vi "Double FFT Mesurament (Max Bin detection - Control - Init Wave&Window - Snapshot - DoubleFFT - Latency - Low Freq) RT Test.vi"() -> ()   [LabVIEW 2014]
uses:
  <vilib>/Platform/TimedLoop/XDataNode/timing_clust.ctl
  <vilib>/Platform/TimedLoop/XDataNode/nitl_modes.ctl
  <vilib>/Platform/TimedLoop/XDataNode/wakeup.ctl
  <vilib>/FPGAPlugInAG/sbRIO-9636/niLvFpga_Open_sbRIO-9636.vi
  <vilib>/rvi/interface/common/dynamic/niFpgaDynamicAddResources.vi
  <vilib>/Utility/error.llb/Error Cluster From Error Code.vi
  <vilib>/rvi/errors/niLvFpgaAdjustHostInterfaceError.vi
  <vilib>/rvi/interface/common/niFpgaWaitOnOcc.vi
  <vilib>/FPGAPlugInAG/Dynamic/niLvFpga_Run_Dynamic.vi
  <vilib>/FPGAPlugInAG/Dynamic/niLvFpga_Abort_Dynamic.vi
  <vilib>/FPGAPlugInAG/Dynamic/niLvFpga_Reset_Dynamic.vi
  <vilib>/FPGAPlugInAG/Dynamic/niLvFpga_Close_Dynamic.vi
  <vilib>/rvi/interface/nirviOpenFPGA/nirviOpenFPGA.xnode
  FPGA Bitfiles/LaserDistanceSen_FPGATarget_DoubleFFTMesuram_ltZoZsQg6NE.lvbitx
  FPGA Target/Test VIs/Double FFT Mesurament (Max Bin detection - Control - Init Wave&Window - Snapshot - DoubleFFT - Latency - Low Freq) test.vi
  <vilib>/rvi/interface/nirviReadWriteControl/nirviReadWriteControl.xnode
  <vilib>/rvi/interface/nirviMethod/nirviMethod.xnode
  <vilib>/Platform/TimedLoop/XDataNode/XDataNode.xnode
  <vilib>/rvi/interface/nirviCloseFPGA/nirviCloseFPGA.xnode
  <vilib>/FPGAPlugInAG/Dynamic/niLvFpga_ConfigureFifo_Dynamic.vi
  <vilib>/rvi/errors/niLvFpgaMergeErrorWithErrorCode.vi
  <vilib>/FPGAPlugInAG/Dynamic/niLvFpga_StartFifo_Dynamic.vi
  <vilib>/rvi/interface/Simulation/niFpgaSimulationCallBeginRW.vi
  <vilib>/FPGAPlugInAG/Dynamic/niLvFpga_ReadFifo_Dynamic.vi
  <vilib>/Platform/TimedLoop/XDataNode/XDNodeRunTimeDep.lvlib
  NiFpgaLv.dll
panel:
  out "maxbin_secondFFT":i32
  out "maxbin_firstFFT":i32
  out "F_rise":dbl
  out "f_fall":dbl
  out "f_mean":dbl
  out "Velocity (m/s)":dbl
  out "Distance (m)":dbl
  in  "Initial Latency points":u32(slide)=10 scale=0.0..1249.0
  out "Second FFT (bin)":dbl[](graph)
  out "Second Signal (points) - Rising Triangular":dbl[](graph)
  out "Elements Remaining FFT":u32
  out "Elements Remaining Signal":u32
  out "First FFT (bin)":dbl[](graph)
  out "First Signal (points) - Falling Triangular":dbl[](graph)
  in  "Snapshot":bool
  in  "Windowing":T1(ring)
  in  "first bin":i32=15
  in  "last bin":i32=255
  in  "lower limit 2":u32(slide)=725 scale=625.0..738.0
  in  "lower limit 1":u32(slide)=100 scale=0.0..113.0
  out "Detected Frequency Tone - (Hz)":dbl
  in  "stop":bool
  out "Max Bin":i32
  out "Max Amp":dbl format="%.2f"
  out "Prev Bin":i32
  out "Next Bin":i32
  out "Prev Amp":dbl format="%.2f"
  out "Next Amp":dbl format="%.2f"
  out "Interpolated Bin":dbl
  in  "Interpolation Method":T2(ring)=enum."Jain"
  # "WARNING:\nOnce pressed wait untill the end of operation"
  # "ONLINE parameter"
  # "OFFLINE parameters"
  # "Max Detection FFT bin range"
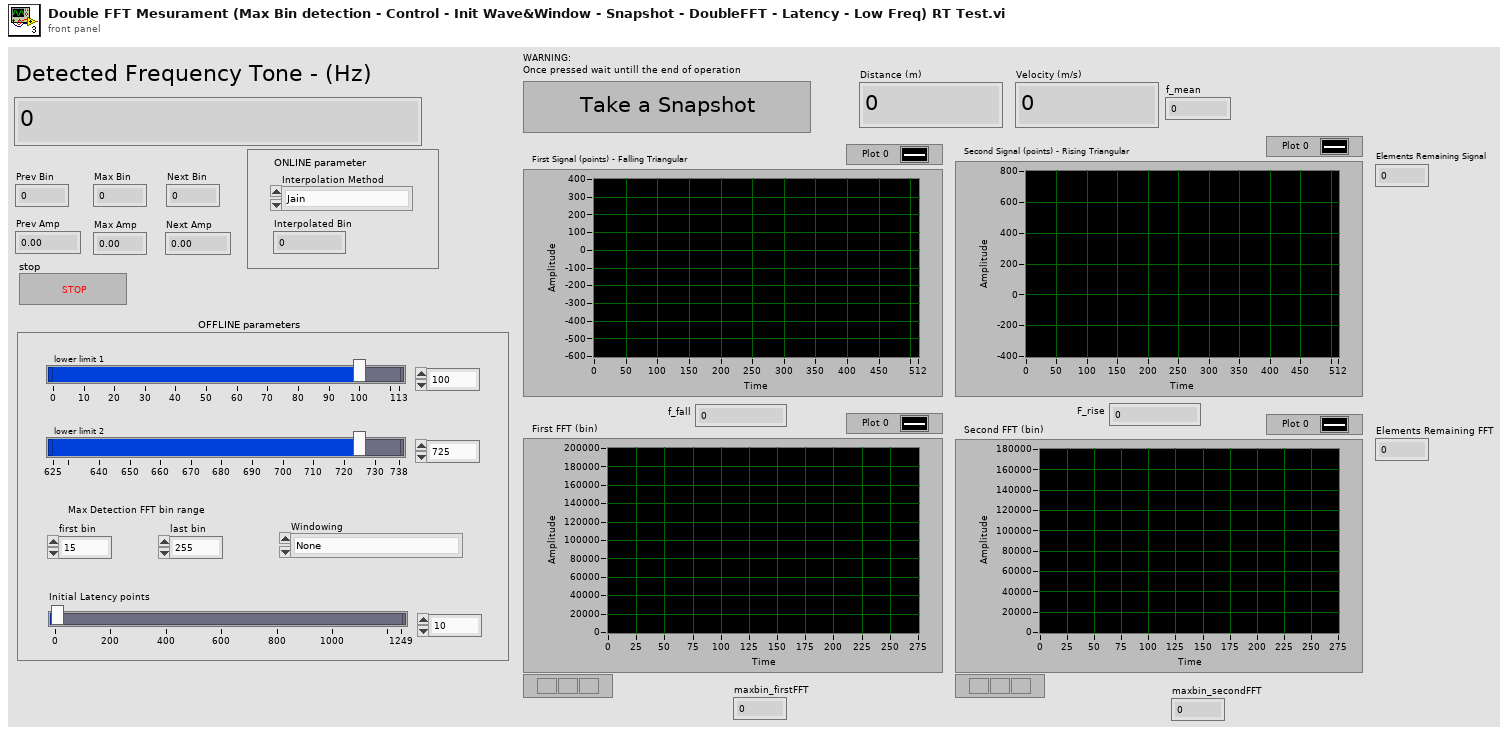
[diagram p1: front panel]
types:
  T1 = enum16{"None", "Hanning", "Hamming", "Blackman", "Blackman-Harris"}
  T2 = enum16{"Quadratic", "McLeodd", "Barycentric", "Jain"}
  T3 = typedef "XDNodeRunTimeDep.lvlib/timing_clust.ctl" = cluster{"Expected End [f-1]":u64, "Actual End [f-1]":u64, "Finished Late? [f-1]":bool, "Expected End [i-1]":u64, "Actual End [i-1]":u64, "Finished Late? [i-1]":bool, "Expected Start [i]":u64, "Actual Start [i]":u64, "Expected Start [f]":u64, "Actual Start [f]":u64, "Source Name":string, "Structure Name":string, "Period":i64, "Deadline":i64, "Offset":i64, "Start":i64, "Priority":i32, "Timeout":i32, "Mode":T4, "Wakeup Reason":T5, "Error":errorcluster, "Source Type":string, "Secondary Source Type":string, "Global End Time":u64, "Global Start Time":u64, "Frame Duration":u64, "Iteration Duration":u64, "Assigned CPU":i32, "I/O Scan Engine Mode":u32}
  T4 = typedef "XDNodeRunTimeDep.lvlib/nitl_modes.ctl" = enum32{"No Change", "Process missed periods, maintain original phase", "Discard missed periods, maintain original phase", "Process missed periods, ignore original phase", "Discard missed periods, ignore original phase"}
  T5 = typedef "XDNodeRunTimeDep.lvlib/wakeup.ctl" = enum32{"Normal", "Aborted", "Asynchronous wakeup", "Timing source error", "Timed loop error", "Timeout"}
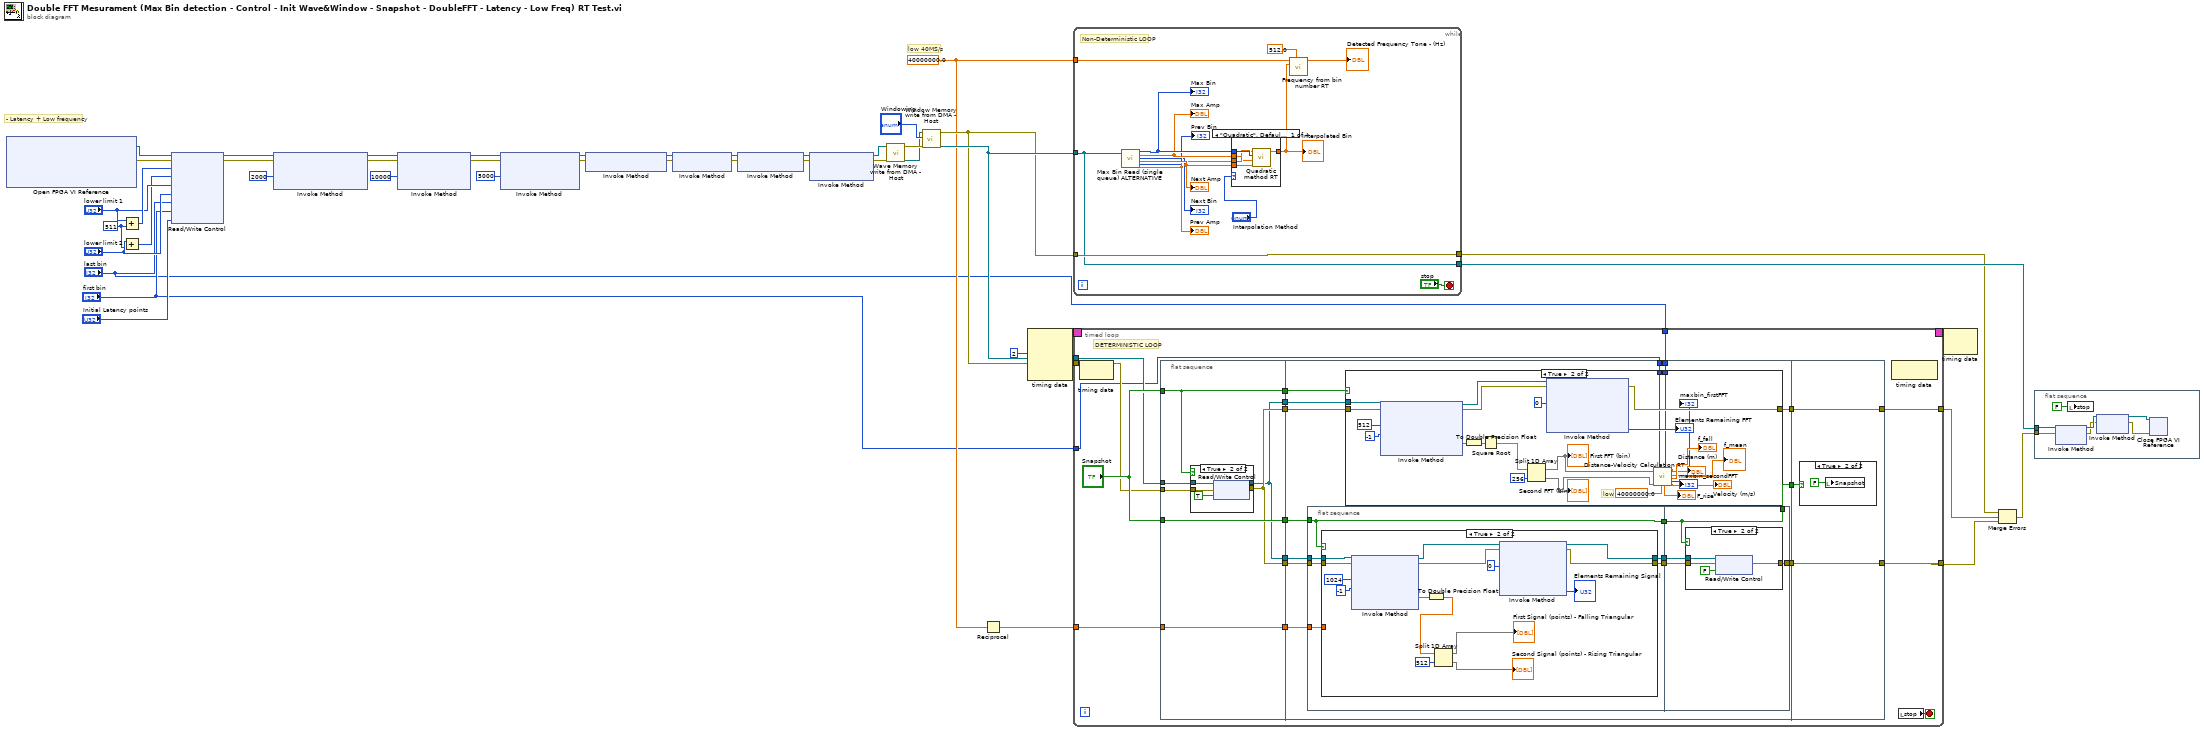
[diagram p0: block diagram]
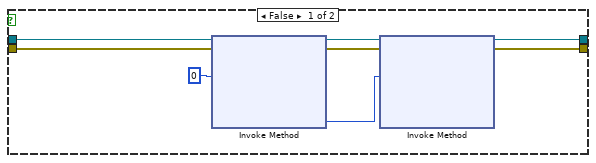
[diagram p3: hidden frame]
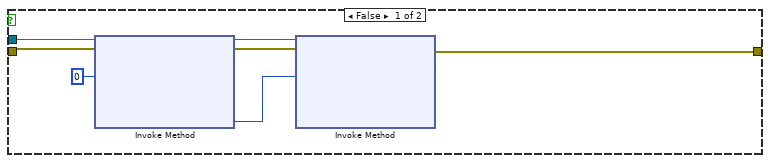
[diagram p5: hidden frame]
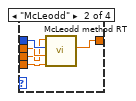
[diagram p7: hidden frame]
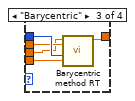
[diagram p8: hidden frame]
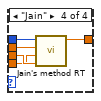
[diagram p9: hidden frame]
diagram:
  w40 = u32 511 ("y")
  w18 = 40000000.0 ("Sample Rate (S/s)")
  # "- Latency + Low frequency"
  # "low 40MS/s"
  n1 = xnode "Open FPGA VI Reference"() -> ("FPGA VI Reference Out"=w39:refnum<k20>, "error out"=w38:errorcluster)  [unwired: 2 in]
  n2 = Add(x="lower limit 1", y=w40) -> (x+y=w44:u32)
  n3 = Add(x="lower limit 2", y=w40) -> (x+y=w42:u32)
  n4 = xnode "Read/Write Control"("FPGA VI Reference In"=w39, "error in"=w38, "upper limit 1"=w44, "upper limit 2"=w42, "lower limit 1"="lower limit 1", "lower limit 2"="lower limit 2", "last bin"="last bin", "first bin"="first bin", "Latency points"="Initial Latency points") -> ("FPGA VI Reference Out"=w33:refnum<k20>, "error out"=w32:errorcluster)
  n5 = xnode "Invoke Method"("FPGA VI Reference In"=w33, "error in"=w32, "Requested Depth"=u32 2000) -> ("FPGA VI Reference Out"=w31:refnum<k20>, "error out"=w30:errorcluster)  [unwired: 1 out]
  n6 = xnode "Invoke Method"("FPGA VI Reference In"=w31, "error in"=w30, "Requested Depth"=u32 10000) -> ("FPGA VI Reference Out"=w29:refnum<k20>, "error out"=w28:errorcluster)  [unwired: 1 out]
  n7 = xnode "Invoke Method"("FPGA VI Reference In"=w29, "error in"=w28, "Requested Depth"=u32 5000) -> ("FPGA VI Reference Out"=w12:refnum<k20>, "error out"=w13:errorcluster)  [unwired: 1 out]
  n8 = xnode "Invoke Method"("FPGA VI Reference In"=w12, "error in"=w13) -> ("FPGA VI Reference Out"=w22:refnum<k20>, "error out"=w21:errorcluster)
  n9 = xnode "Invoke Method"("FPGA VI Reference In"=w22, "error in"=w21) -> ("FPGA VI Reference Out"=w24:refnum<k20>, "error out"=w23:errorcluster)
  n10 = xnode "Invoke Method"("FPGA VI Reference In"=w24, "error in"=w23) -> ("FPGA VI Reference Out"=w10:refnum<k20>, "error out"=w11:errorcluster)
  n11 = xnode "Invoke Method"("FPGA VI Reference In"=w10, "error in"=w11) -> ("FPGA VI Reference Out"=w17:refnum<k20>, "error out"=w16:errorcluster)  [unwired: 1 in]
  n12 = call "Wave Memory write from DMA - Host.vi"("error in"=w16, "FPGA VI Reference In"=w17) -> ("FPGA VI Reference Out"=w14:refnum<k20>, "error out"=w15:errorcluster)  [unwired: 7 in, 1 out]
  n13 = call "Window Memory write from DMA - Host.vi"("error in"=w15, "Enum"="Windowing", "FPGA VI Reference In"=w14) -> ("FPGA VI Reference Out"=w35:refnum<k20>, "error out"=w34:errorcluster)  [unwired: 5 in, 2 out]
  n14 = Reciprocal(x=w18) -> (1/x=w19:dbl)
  n15 = node-c288(i64 2 ("Period")) -> (w9:T3)  [unwired: 3 in]
  n16 = while {
    tunnel: w18 -> [w57]
    tunnel: w35 -> [w55]
    tunnel: w34 -> [w56]
    tunnel: [w55] -> w37
    tunnel: [w56] -> w5
    stop <- "stop" stop-if-true
    # "Non-Deterministic LOOP"
    n17 = call "Max Bin Read (single queue) ALTERNATIVE.vi"("FPGA VI Reference In"=w55) -> ("Max Bin"=w51:i32, "Max Amp"=w50:dbl, "Next Bin"=→"Next Bin":i32, "Next Amp"=w49:dbl, "Prev Bin"=→"Prev Bin":i32, "Prev Amp"=w48:dbl)  [unwired: 12 in, 1 out]
    "Max Bin" <- w51
    "Max Amp" <- w50
    "Prev Amp" <- w48
    "Next Amp" <- w49
    n18 = case shown="\"Quadratic\", Default" "Interpolation Method" {
      tunnel: w51 -> [w62 w67 w72 w77]
      tunnel: w50 -> [w59 w66 w71 w76]
      tunnel: w48 -> [w60 w65 w70 w75]
      tunnel: w49 -> [w61 w64 w69 w74]
      tunnel: [w63 w68 w73 w78] -> w52
      frame "Quadratic", Default {
        n19 = call "Quadratic method RT.vi"("Next Amplitude"=w61, "Max Amplitude"=w59, "Max bin"=w62, "Prev Amplitude"=w60) -> ("Bin"=w63:dbl)  [unwired: 7 in]
      }
      frame "McLeodd" {
        n20 = call "McLeodd method RT.vi"("Next Amp"=w64, "Max Amp"=w66, "Max Bin"=w67, "Prev Amp"=w65) -> ("Bin"=w68:dbl)  [unwired: 7 in]
      }
      frame "Barycentric" {
        n21 = call "Barycentric method RT.vi"("Next Amp"=w69, "Max Bin"=w72, "Max Amp"=w71, "Prev Amp"=w70) -> ("Bin"=w73:dbl)  [unwired: 7 in]
      }
      frame "Jain" {
        n22 = call "Jain's method RT.vi"("Prev Amp"=w75, "Next Amp"=w74, "Max Amp"=w76, "Max Bin"=w77) -> ("Bin"=w78:dbl)  [unwired: 7 in]
      }
    }
    "Interpolated Bin" <- w52
    n23 = call "Frequency from bin number RT.vi"("FFT size"=512.0, "Bin number"=w52, "Sample Rate (S/s)"=w57) -> ("Detected Frequency (Hz)"=→"Detected Frequency Tone - (Hz)":dbl)  [unwired: 8 in]
  }
  n24 = timed-loop {
    tunnel: w35 -> [w91]
    tunnel: w34 -> [w92]
    tunnel: [w94] -> w6
    tunnel: w19 -> [w96]
    tunnel: [w95] -> w4
    timing: w9 -> [_]
    timing-out: [_] -> w8
    tunnel: "first bin" -> [w80]
    tunnel: "last bin" -> [w79]
    stop <- w97 stop-if-true
    # "DETERMINISTIC LOOP"
    n25 = node-c288() -> ()  [unwired: 1 in, 1 out]
    n26 = flat-sequence {
      tunnel: w91 -> [w102]
      tunnel: w92 -> [w103]
      tunnel: "Snapshot" -> [w100]
      tunnel: "Snapshot" -> [w105]
      tunnel: w96 -> [w106]
      tunnel: [w104] -> w90
      tunnel: [w106] -> w89
      tunnel: [w105] -> w88
      tunnel: [w100] -> w87
      tunnel: [w104] -> w86
      tunnel: [w101] -> w85
      tunnel: [w101] -> w84
      tunnel: w90 -> [w124]
      tunnel: w89 -> [w123]
      tunnel: w88 -> [w117]
      tunnel: w87 -> [w120]
      tunnel: w86 -> [w119]
      tunnel: w85 -> [w118]
      tunnel: w84 -> [w125]
      tunnel: [w122] -> w83
      tunnel: [w121] -> w82
      tunnel: [w116] -> w81
      tunnel: w80 -> [w115]
      tunnel: w79 -> [w114]
      tunnel: [w200] -> w94
      tunnel: [w201] -> w95
      tunnel: w83 -> [w201]
      tunnel: w82 -> [w200]
      tunnel: w81 -> [w199]
      frame #0 {
        n27 = case shown="True" w100 {
          tunnel: [w107 w112] -> w104
          tunnel: w103 -> [w107 w111]
          tunnel: w102 -> [w108 w110]
          tunnel: [w108 w109] -> w101
          frame False {
          }
          frame True {
            n28 = xnode "Read/Write Control"("FPGA VI Reference In"=w110, "error in"=w111, "snapshot"=TRUE) -> ("FPGA VI Reference Out"=w109:refnum<k20>, "error out"=w112:errorcluster)
          }
        }
      }
      frame #1 {
        n29 = flat-sequence {
          tunnel: w125 -> [w134]
          tunnel: w124 -> [w133]
          tunnel: w123 -> [w132]
          tunnel: w117 -> [w129]
          tunnel: [w131] -> w128
          tunnel: [w130] -> w127
          tunnel: [w129] -> w126
          tunnel: [w159] -> w121
          tunnel: w128 -> [w161]
          tunnel: w127 -> [w160]
          tunnel: w126 -> [w158]
          tunnel: [w158] -> w116
          frame #0 {
            n30 = case shown="True" w129 {
              tunnel: w134 -> [w141 w157]
              tunnel: w133 -> [w139 w156]
              tunnel: [w138 w149] -> w130
              tunnel: w132 -> [_ _]
              tunnel: [w135 w148] -> w131
              frame False {
                n31 = xnode "Invoke Method"("FPGA VI Reference In"=w141, "error in"=w139, "Number of Elements"=u32 0) -> ("FPGA VI Reference Out"=w137:refnum<k20>, "error out"=w136:errorcluster, "Elements Remaining"=w140:u32)  [unwired: 1 in, 1 out]
                n32 = xnode "Invoke Method"("FPGA VI Reference In"=w137, "error in"=w136, "Number of Elements"=w140) -> ("FPGA VI Reference Out"=w135:refnum<k20>, "error out"=w138:errorcluster)  [unwired: 1 in, 2 out]
              }
              frame True {
                n33 = xnode "Invoke Method"("FPGA VI Reference In"=w157, "error in"=w156, "Number of Elements"=u32 1024, "Timeout (ms)"=-1) -> ("FPGA VI Reference Out"=w151:refnum<k20>, "error out"=w150:errorcluster, "Data"=w153:fxp<+/-,12,12>[])  [unwired: 1 out]
                n34 = To Double Precision Float(number=w153) -> (double precision float=w146:dbl[])
                n35 = Split 1D Array(array=w146, index=512) -> (first subarray=→"First Signal (points) - Falling Triangular":dbl[], second subarray=→"Second Signal (points) - Rising Triangular":dbl[])
                n36 = xnode "Invoke Method"("FPGA VI Reference In"=w151, "error in"=w150, "Number of Elements"=u32 0) -> ("FPGA VI Reference Out"=w148:refnum<k20>, "error out"=w149:errorcluster, "Elements Remaining"=→"Elements Remaining Signal":u32)  [unwired: 1 in, 1 out]
              }
            }
          }
          frame #1 {
            n37 = case shown="True" w158 {
              tunnel: [w162 w164] -> w159
              tunnel: w161 -> [_ w165]
              tunnel: w160 -> [w162 w163]
              frame False {
              }
              frame True {
                n38 = xnode "Read/Write Control"("FPGA VI Reference In"=w165, "error in"=w163, "snapshot"=FALSE) -> ("error out"=w164:errorcluster)  [unwired: 1 out]
              }
            }
          }
        }
        n39 = case shown="True" w120 {
          tunnel: w118 -> [w172 w193]
          tunnel: w119 -> [w169 w194]
          tunnel: [w168 w192] -> w122
          tunnel: w115 -> [_ w176]
          tunnel: w114 -> [_ w177]
          frame False {
            n40 = xnode "Invoke Method"("FPGA VI Reference In"=w172, "error in"=w169, "Number of Elements"=u32 0) -> ("FPGA VI Reference Out"=w170:refnum<k20>, "error out"=w167:errorcluster, "Elements Remaining"=w171:u32)  [unwired: 1 in, 1 out]
            n41 = xnode "Invoke Method"("FPGA VI Reference In"=w170, "error in"=w167, "Number of Elements"=w171) -> ("error out"=w168:errorcluster)  [unwired: 1 in, 3 out]
          }
          frame True {
            # "low"
            n42 = xnode "Invoke Method"("FPGA VI Reference In"=w193, "error in"=w194, "Number of Elements"=u32 512, "Timeout (ms)"=-1) -> ("FPGA VI Reference Out"=w190:refnum<k20>, "error out"=w191:errorcluster, "Data"=w196:fxp<+,44,44>[])  [unwired: 1 out]
            n43 = To Double Precision Float(number=w196) -> (double precision float=w195:dbl[])
            n44 = Square Root(x=w195) -> (sqrt(x)=w187:dbl[])
            n45 = Split 1D Array(array=w187, index=256) -> (first subarray=w185:dbl[], second subarray=w184:dbl[])
            "First FFT (bin)" <- w185
            "Second FFT (bin)" <- w184
            n46 = xnode "Invoke Method"("FPGA VI Reference In"=w190, "error in"=w191, "Number of Elements"=u32 0) -> ("error out"=w192:errorcluster, "Elements Remaining"=→"Elements Remaining FFT":u32)  [unwired: 1 in, 2 out]
            n47 = call "Distance-Velocity Calculation RT.vi"("First FFT"=w185, "Second FFT"=w184, "first FFT bin"=w176, "Sample Rate (S/s)"=40000000.0, "last FFT bin"=w177) -> ("F_rise"=→"F_rise":dbl, "maxbin_firstFFT"=→"maxbin_firstFFT":i32, "maxbin_secondFFT"=→"maxbin_secondFFT":i32, "Distance (m)"=→"Distance (m)":dbl, "f_mean"=→"f_mean":dbl, "F_fall"=→"f_fall":dbl, "Velocity (m/s)"=→"Velocity (m/s)":dbl)  [unwired: 8 in]
          }
        }
      }
      frame #2 {
        n48 = case shown="True" w199 {
          frame False {
          }
          frame True {
            n49 = local write "Snapshot"(FALSE ("Snapshot")) -> ()
          }
        }
      }
    }
    n50 = node-c288() -> ()  [unwired: 1 in, 1 out]
    n51 = local read "stop"() -> (w97:bool)
  }
  n52 = node-c288(w8) -> ()  [unwired: 1 out]
  n53 = Merge Errors(w5, w4, w6) -> (w20:errorcluster)
  n54 = flat-sequence {
    tunnel: w37 -> [w209]
    tunnel: w20 -> [w208]
    frame #0 {
      n55 = xnode "Invoke Method"("FPGA VI Reference In"=w209, "error in"=w208) -> ("FPGA VI Reference Out"=w204:refnum<k20>, "error out"=w203:errorcluster)
      n56 = local write "stop"(FALSE ("stop")) -> ()
      n57 = xnode "Invoke Method"("FPGA VI Reference In"=w204, "error in"=w203) -> ("FPGA VI Reference Out"=w205:refnum<k20>, "error out"=w206:errorcluster)
      n58 = xnode "Close FPGA VI Reference"("FPGA VI Reference In"=w205, "error in"=w206) -> ()  [unwired: 1 out]
    }
  }
